vi "SineGennerateI32.vi"(9 "frequency":dbl=3.0 format="%#_13g", 10 "limit":dbl=40.0 format="%#_13g") -> (2 "x":i32, 3 "y":i32)   [LabVIEW 2018, in "RandomMoveBool.lvclass"]
uses:
  RandomMoveBool.lvclass
panel:
  out "index":dbl
  out "dt":dbl
  out "Y":dbl[](array[numeric])
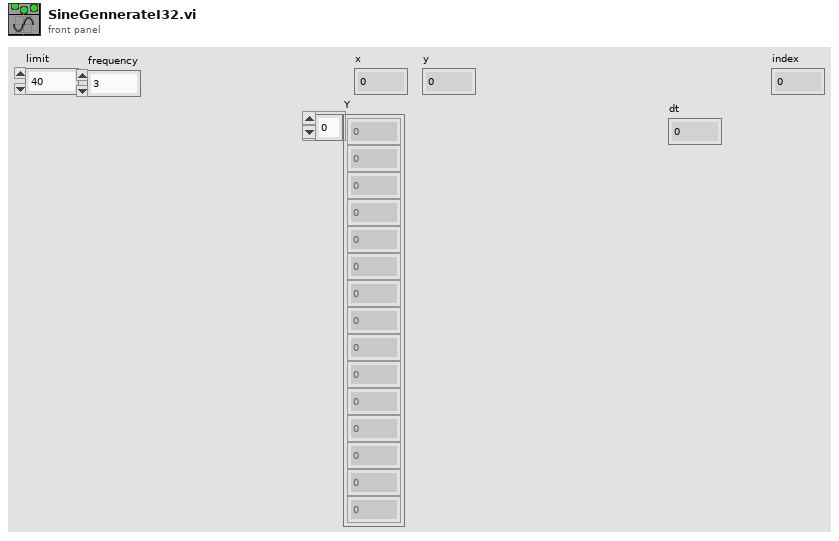
[diagram p1: front panel]
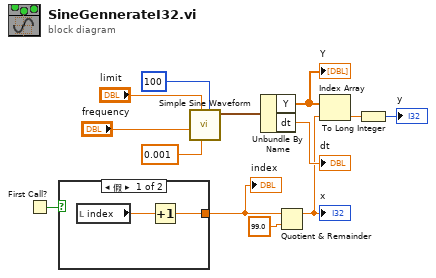
[diagram p0: block diagram]
diagram:
  n1 = First Call?() -> (First Call?: T/F=w8:bool)
  n2 = case shown="假" w8 {
    tunnel: [w14 _] -> w7
    frame False {
      n3 = local read "index"() -> (w15:dbl)
      n4 = Increment(x=w15) -> (x+1=w14:dbl)
    }
    frame True {
    }
  }
  "index" <- w7
  n5 = call "Simple Sine Waveform.vi"("n点"=100 ("n points"), "△t"=0.001 ("delta t"), "幅值"="limit", "n周期"="frequency") -> ("正弦波形"=w5:waveform(dbl))  [unwired: 7 in]
  n6 = Unbundle By Name(w5) -> ("Y"=w10:dbl[], "dt"=→"dt":dbl)
  "Y" <- w10
  n7 = Quotient & Remainder(x=w7, y=99.0) -> (x-y*floor(x/y)=w1:dbl)  [unwired: 1 out]
  "x" <- w1
  n8 = Index Array(array=w10, index=w1) -> (element=w9:dbl)
  n9 = To Long Integer(number=w9) -> (32bit integer=→"y":i32)
